vi "LWXPS_ZygoRegisterSet.vi"(0 "Positioner name":string, 1 "XPS Reference IN":refnum<k24>, 2 "Register value":i32, 3 "Value":i32, 4 "LabVIEW error IN":errorcluster) -> (6 "XPS Reference OUT":refnum<k24>, 7 "Returned error code":i32, 9 "XPS Error String":string, 10 "LabVIEW error OUT":errorcluster)   [LabVIEW 2014]
uses:
  D:/XPSQ8_LabView_Library/Development/Source/Dll/Newport.XPS.CommandInterface.dll
  Dll/Newport.XPS.CommandInterface.dll
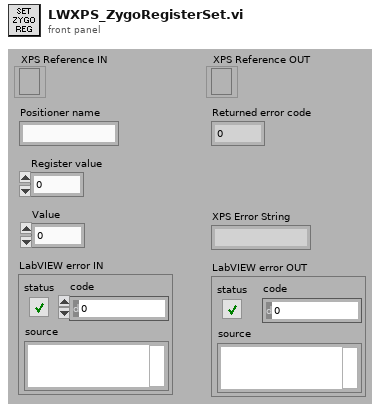
[diagram p1: front panel]
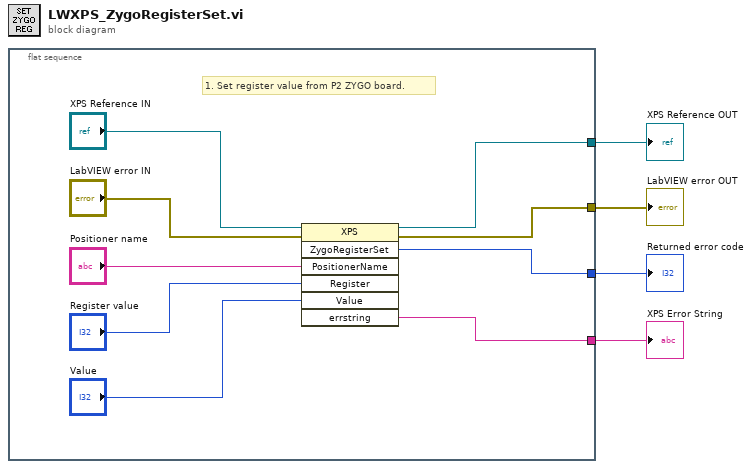
[diagram p0: block diagram]
diagram:
  n1 = flat-sequence {
    tunnel: [w11] -> w4
    tunnel: [w8] -> w3
    tunnel: [w12] -> w2
    tunnel: [w7] -> w1
    frame #0 {
      # "1. Set register value from P2 ZYGO board."
      n2 = invoke class="XPS" method="ZygoRegisterSet"(reference="XPS Reference IN", error in="LabVIEW error IN", "PositionerName"="Positioner name", "Register"="Register value", "Value"="Value") -> (reference out=w11:refnum<k24>, error out=w8:errorcluster, "ZygoRegisterSet"=w12:i32, "errstring"=w7:string)  [unwired: 2 in, 3 out]
    }
  }
  "XPS Reference OUT" <- w4
  "LabVIEW error OUT" <- w3
  "Returned error code" <- w2
  "XPS Error String" <- w1
